vi "rs3 Advanced Set Census Enable Reg3.vi"(8 "error in (no error)":errorcluster, 10 "ST_CensusEnableReg":cluster{"uDiameter":u32, "vDiameter":u32}, 11 "device in":u64) -> (0 "error out":errorcluster, 1 "error":u64, 3 "Dev out":u64)   [LabVIEW 2023]
doc: "Sets registers inside the ASIC that affect the depth calculations"
panel:
  # "RS3 Adv. Set Census Reg"
  # "(C) 2017 Intel Corp.,  AGJ"
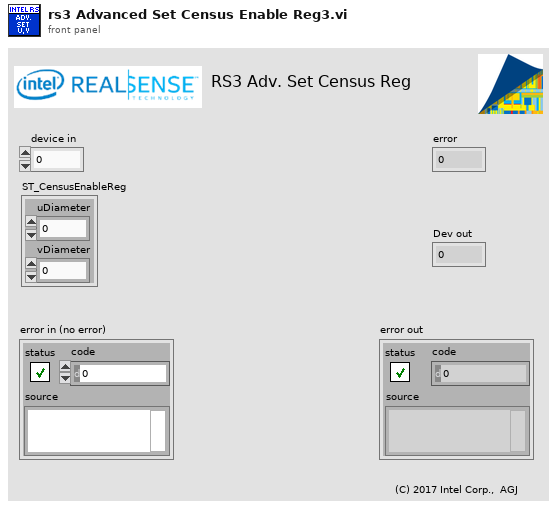
[diagram p1: front panel]
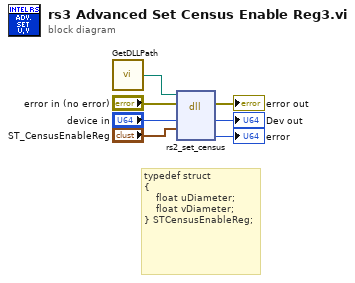
[diagram p0: block diagram]
diagram:
  # "typedef struct\n{\n    float uDiameter;\n    float vDiameter;\n} STCensusEnableReg;"
  n1 = call "GetDLLPath.vi"() -> ("DLL Path"=w1:path)
  n2 = dll-call lib="C:/STEAMSyndicate/RealSenseWrappers/VI Wrappers (add ons) Public/RealSense/realsense2.dll" fn="rs2_set_census"(path in=w1, error in="error in (no error)", "device"="device in", "ST SLO Threshold"="ST_CensusEnableReg") -> (error out=→"error out":errorcluster, "device"=→"Dev out":u64, "error"=→"error":u64)  [unwired: 4 in, 1 out]
